vi "test.vi"(11 "YoutuberDownloader":refnum<class "YoutuberDownloader.lvclass">) -> (0 "error out":errorcluster, 3 "estimatedTime":u32)   [LabVIEW 2017, in "Demo.lvclass"]
uses:
  Demo.lvclass
  YoutuberDownloader Class/YoutuberDownloader.lvclass
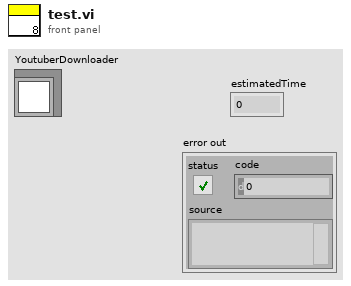
[diagram p1: front panel]
types:
  T1 = enum16{"Create", "Get Reference", "Print", "Close"}
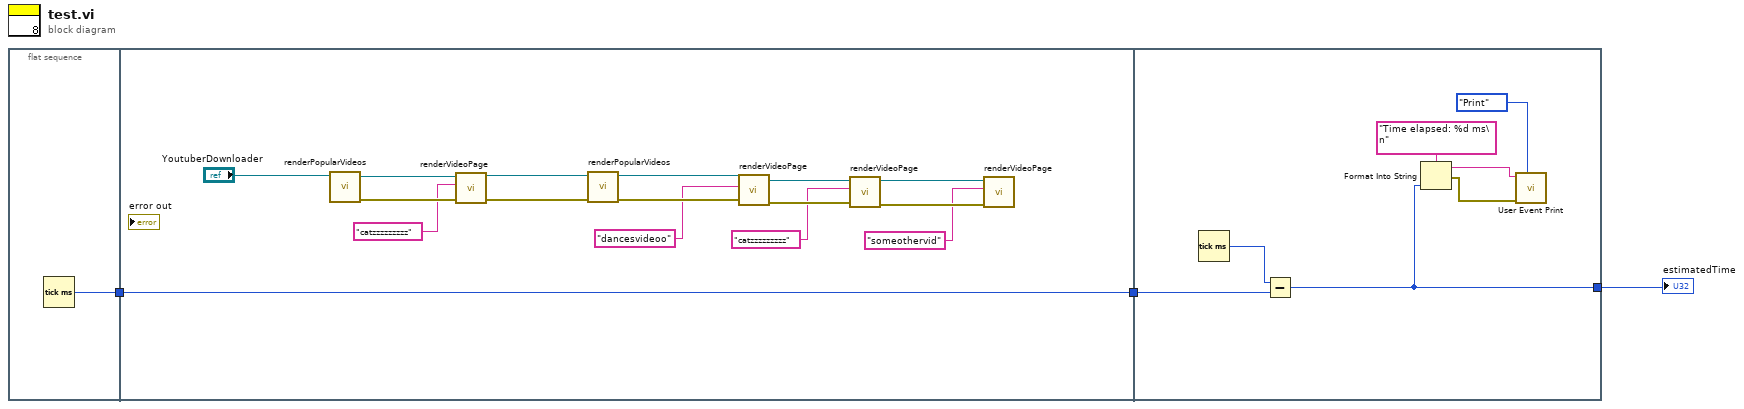
[diagram p0: block diagram]
diagram:
  n1 = flat-sequence {
    tunnel: [w4] -> w3
    tunnel: w3 -> [w5]
    tunnel: [w5] -> w2
    tunnel: w2 -> [w26]
    tunnel: [w24] -> w1
    frame #0 {
      n2 = Tick Count (ms)() -> (millisecond timer value=w4:u32)
    }
    frame #1 {
      n3 = call "renderPopularVideos.vi"("YoutuberDownloader in"="YoutuberDownloader") -> ("error out"=w18:errorcluster, "YoutuberDownloader out"=w19:refnum<class "YoutuberDownloader.lvclass">)  [unwired: 9 in]
      n4 = call "renderVideoPage.vi"("error in (no error)"=w18, "VideoId"="catzzzzzzzzz", "YoutuberDownloader in"=w19) -> ("error out"=w15:errorcluster, "YoutuberDownloader out"=w16:refnum<class "YoutuberDownloader.lvclass">)  [unwired: 7 in]
      n5 = call "renderPopularVideos.vi"("error in (no error)"=w15, "YoutuberDownloader in"=w16) -> ("error out"=w13:errorcluster, "YoutuberDownloader out"=w14:refnum<class "YoutuberDownloader.lvclass">)  [unwired: 8 in]
      n6 = call "renderVideoPage.vi"("error in (no error)"=w13, "VideoId"="dancesvideoo", "YoutuberDownloader in"=w14) -> ("error out"=w8:errorcluster, "YoutuberDownloader out"=w9:refnum<class "YoutuberDownloader.lvclass">)  [unwired: 7 in]
      n7 = call "renderVideoPage.vi"("error in (no error)"=w8, "VideoId"="catzzzzzzzzz", "YoutuberDownloader in"=w9) -> ("error out"=w10:errorcluster, "YoutuberDownloader out"=w11:refnum<class "YoutuberDownloader.lvclass">)  [unwired: 7 in]
      n8 = call "renderVideoPage.vi"("error in (no error)"=w10, "VideoId"="someothervid", "YoutuberDownloader in"=w11) -> ()  [unwired: 7 in, 2 out]
    }
    frame #2 {
      n9 = Tick Count (ms)() -> (millisecond timer value=w27:u32)
      n10 = Subtract(x=w27, y=w26) -> (x-y=w24:u32)
      n11 = Format Into String(format string="Time elapsed: %d ms\n", w24) -> (resulting string=w23:string, error out=w22:errorcluster)  [unwired: 2 in]
      n12 = call "User Event Print.vi"("Options"=T1."Print", "error in (no error)"=w22, "String to Print"=w23) -> ()  [unwired: 7 in, 2 out]
    }
  }
  "estimatedTime" <- w1
